vi "Read Mediator Ref.vi"(11 "IController in":refnum<class "IController.lvclass">) -> (2 "Mediator Enququer":refnum<class "Message Enqueuer.lvclass">)   [LabVIEW 2015, in "IController.lvlib" / "IController.lvclass"]
uses:
  IController.lvclass
  <vilib>/ActorFramework/Message Enqueuer/Message Enqueuer.lvclass
  IController.lvclass/IController.ctl
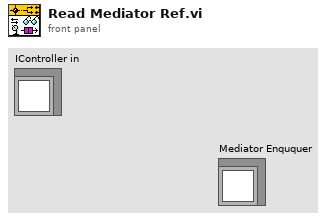
[diagram p1: front panel]
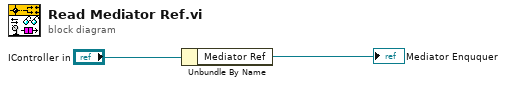
[diagram p0: block diagram]
diagram:
  n1 = Unbundle By Name("IController in") -> ("Mediator Ref"=→"Mediator Enququer":refnum<class "Message Enqueuer.lvclass">)
